vi "Write.vi"(8 "error in (no error)":errorcluster, 10 "Cluster Array":variant, 11 "Cluster Array in":refnum<class "Cluster Array.lvclass">) -> (0 "error out":errorcluster, 1 "Success?":bool, 3 "Cluster Array out":refnum<class "Cluster Array.lvclass">)   [LabVIEW 2020, in "Data.lvlib" / "Cluster Array.lvclass"]
doc: "Write Cluster Array."
uses:
  Cluster Array.lvclass
  Cluster Array.lvclass/Cluster Array.ctl
  Cluster/Cluster.lvclass
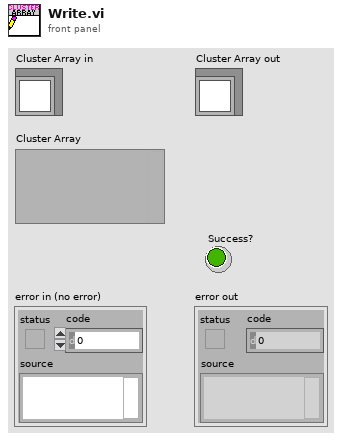
[diagram p1: front panel]
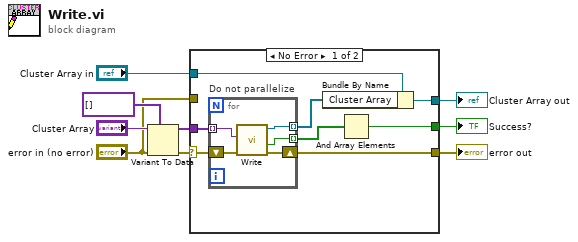
[diagram p0: block diagram]
diagram:
  n1 = Variant To Data(error in="error in (no error)", type=variant[] [] ("Cluster Array"), Variant="Cluster Array") -> (data=w2:variant[], error out=w4:errorcluster)
  n2 = case shown="No Error" w4 {
    selector: w4 -> [w10 _]
    tunnel: [w13 w23] -> w9
    tunnel: [w16 w24] -> w7
    tunnel: "Cluster Array in" -> [w17 w24]
    tunnel: "error in (no error)" -> [_ w23]
    tunnel: w2 -> [w15 _]
    tunnel: [w11 _] -> w1
    frame No Error {
      n3 = for "Do not parallelize" {
        tunnel: w15 -> [w22] mode=indexing
        tunnel: [w19] -> w12 mode=indexing
        tunnel: [w18] -> w14 mode=indexing
        shift-right: [w20] -> w13
        shift-left: w10 -> [w21]
        n4 = call "Write.vi"("error in (no error)"=w21, "Cluster"=w22) -> ("error out"=w20:errorcluster, "Success?"=w19:bool, "Cluster out"=w18:refnum<class "Cluster.lvclass">)  [unwired: 7 in]
      }
      n5 = Bundle By Name(cluster=w17, "Cluster Array"=w14) -> (w16:refnum<class "Cluster Array.lvclass">)
      n6 = And Array Elements(Boolean array=w12) -> (logical AND=w11:bool)
    }
    frame Error {
    }
  }
  "error out" <- w9
  "Cluster Array out" <- w7
  "Success?" <- w1
